vi "Ctor.vi"(8 "error in (no error)":errorcluster, 11 "ExBlank in":refnum<class "ExBlank.lvclass">) -> (0 "error out":errorcluster, 3 "ExBlank out":refnum<class "ExBlank.lvclass">)   [LabVIEW 2020, in "2D Array Example.lvlib" / "ExBlank.lvclass"]
uses:
  ExBlank.lvclass
  ExBlank.lvclass/ExBlank.ctl
  OOPanel/2DPanelBlank/2DPanelBlank.lvclass
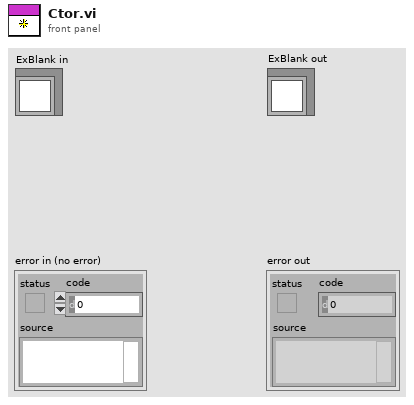
[diagram p1: front panel]
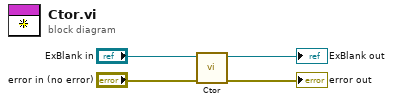
[diagram p0: block diagram]
diagram:
  n1 = call-parent "Ctor.vi"("error in (no error)"="error in (no error)", "ArrayPanel in"="ExBlank in") -> ("error out"=→"error out":errorcluster, "ArrayPanel out"=→"ExBlank out":refnum<class "ExBlank.lvclass">)  [unwired: 8 in]
